vi "OA Get String.vi"(7 "uiStringLen":u32, 8 "error in (no error)":errorcluster, 9 "pcStringValue":string, 10 "pcModeParam":string, 11 "pcModeName":string) -> (0 "error out":errorcluster, 1 "pcStringValue out":string, 3 "function return":u32)   [LabVIEW 2014, in "atmcd32d.lvlib"]
doc: "unsigned int WINAPI OA_GetString(const char * const pcModeName, const char * const pcModeParam, char * pcStringValue, const unsigned int uiStringLen);"
uses:
  atmcd32d.lvlib
  atmcd32d.dll
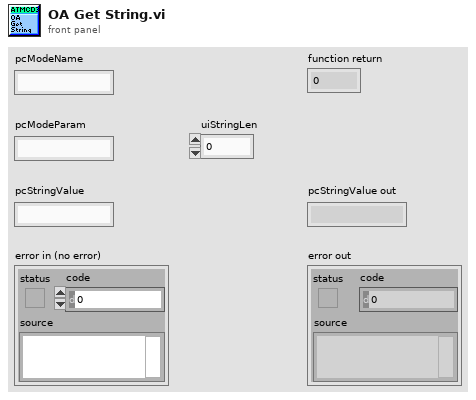
[diagram p1: front panel]
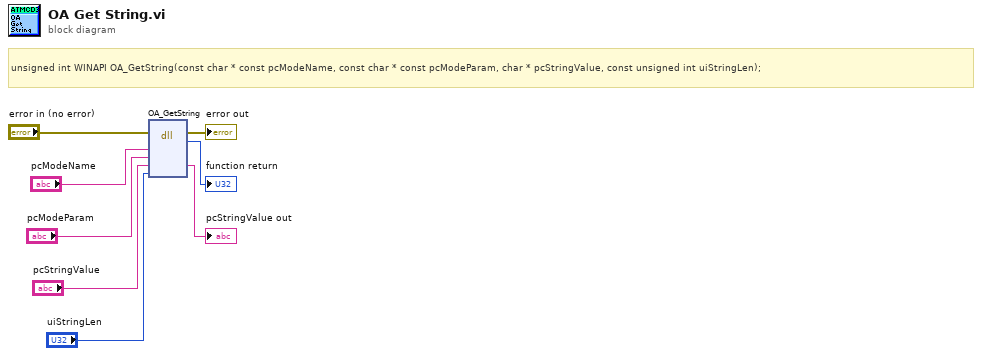
[diagram p0: block diagram]
diagram:
  # "unsigned int WINAPI OA_GetString(const char * const pcModeName, const char * const pcModeParam, char * pcStringValue, const unsigned int uiStringLen);"
  n1 = dll-call lib="C:/Users/Bakir/Documents/Lambda2-Testing/lib/Andorlib/atmcd32d.*" fn="OA_GetString"(error in="error in (no error)", "pcModeName"="pcModeName", "pcModeParam"="pcModeParam", "pcStringValue"="pcStringValue", "uiStringLen"="uiStringLen") -> (error out=→"error out":errorcluster, →"function return":u32, "pcStringValue"=→"pcStringValue out":string)  [unwired: 5 in, 1 out]
